vi "uc480_SimpleLive_Memory_Sequence.vi"() -> ()   [LabVIEW 2011]
uses:
  C:/Program Files/Thorlabs/Scientific Imaging/DCx Camera Support/Develop/DotNet/uc480DotNet.dll
  Develop/DotNet/uc480DotNet.dll
panel:
  out "Acquisition":picture
  in  "Active \nAcquisition Buffer":i32 min=0 max=2 step=1
  in  "Active \nOutput Buffer":u32 max=2 step=1
  in  "Num Buffers":i32=2 min=0 max=100 step=1
  out "Output":picture
  in  "Camera ID":i32
  out "Serial Number":string
  out "AOI Height":i32=8
  out "AOI Width":i32=8
  out "Bits/Pixel":i32=8
  out "Error Out":errorcluster caption="error"
  in  "Exit Camera":bool
  in  "Init Camera":bool
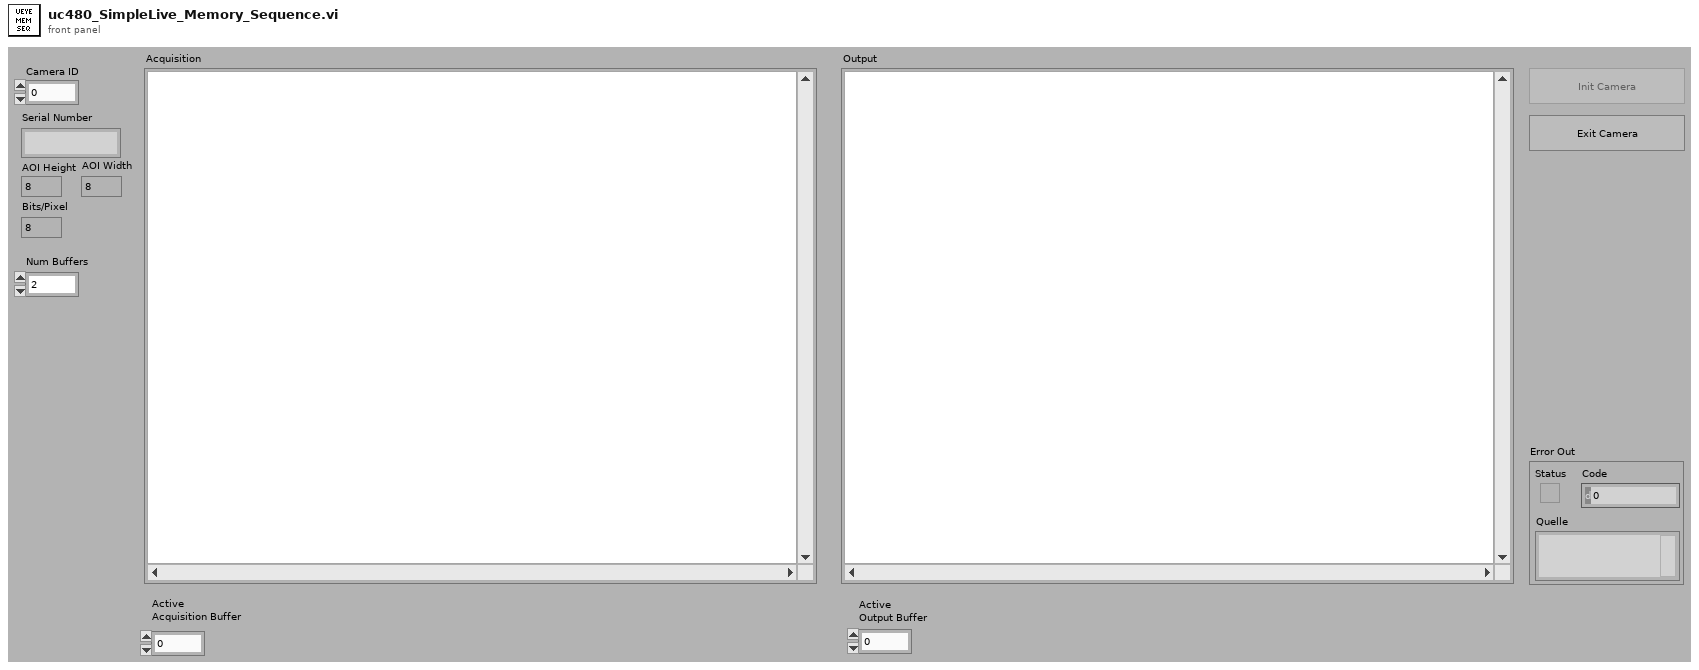
[diagram p1: front panel]
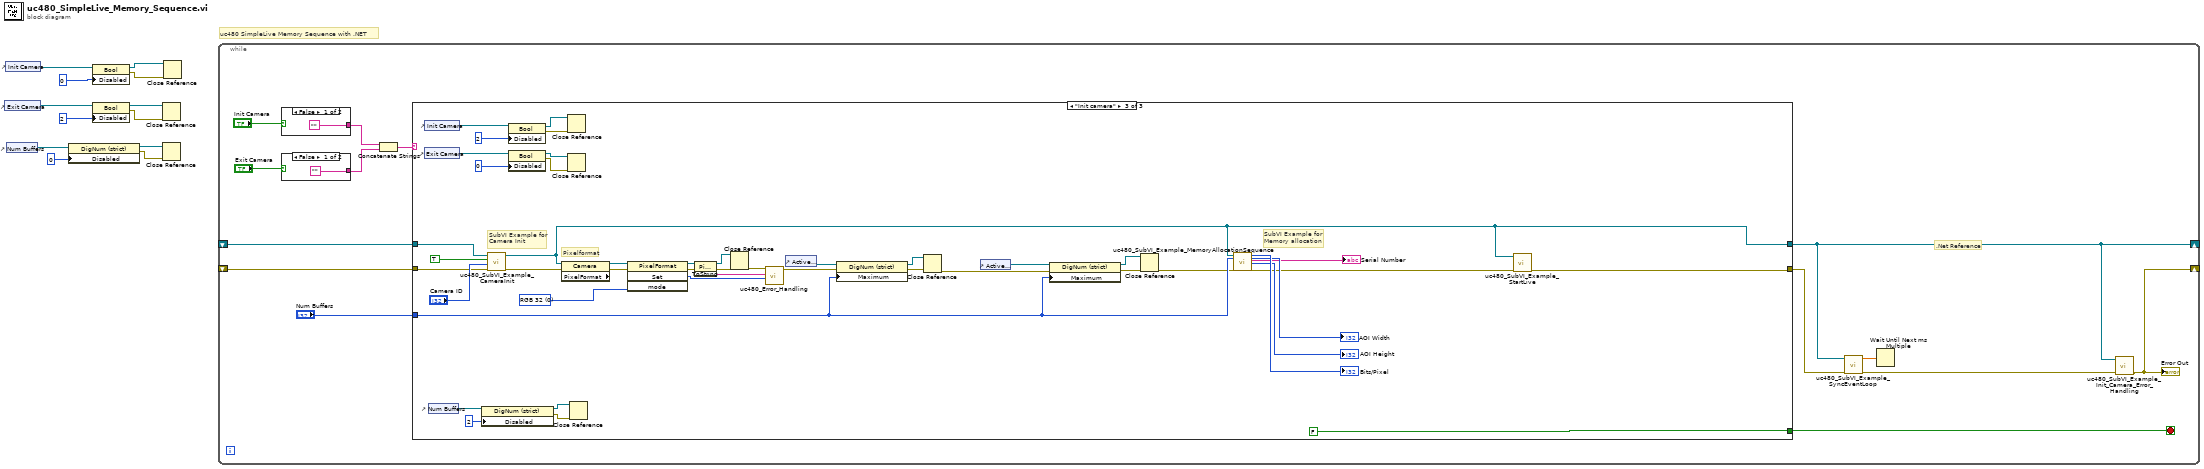
[diagram p0: block diagram]
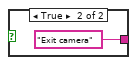
[diagram p2: hidden frame]
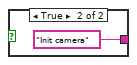
[diagram p3: hidden frame]
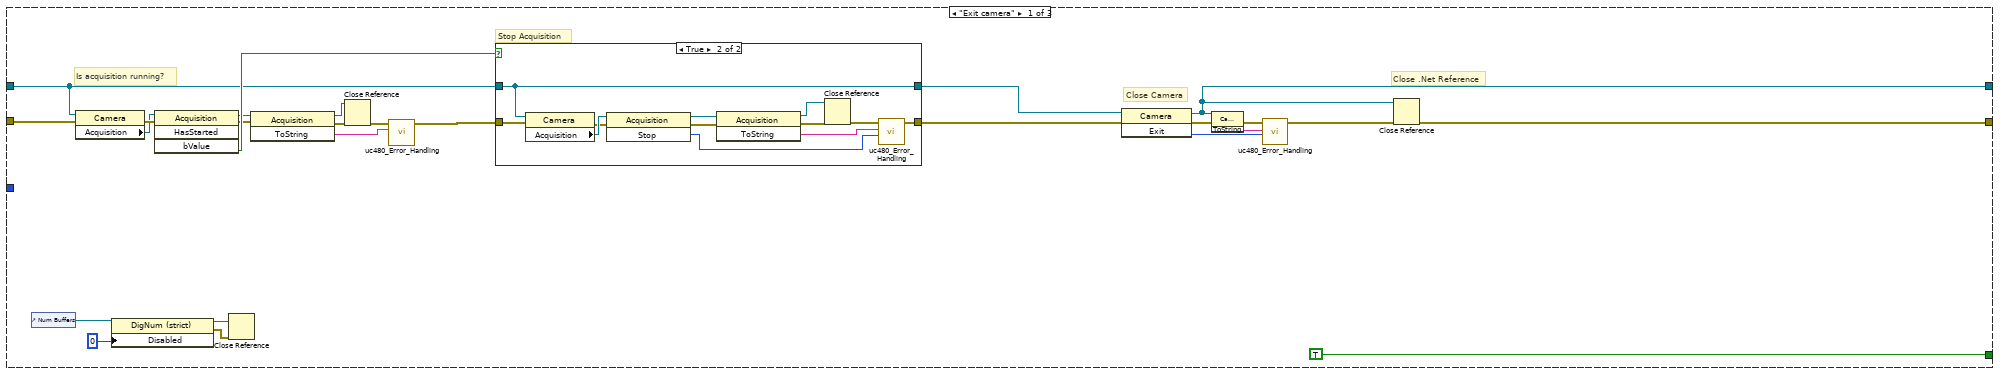
[diagram p4: hidden frame]
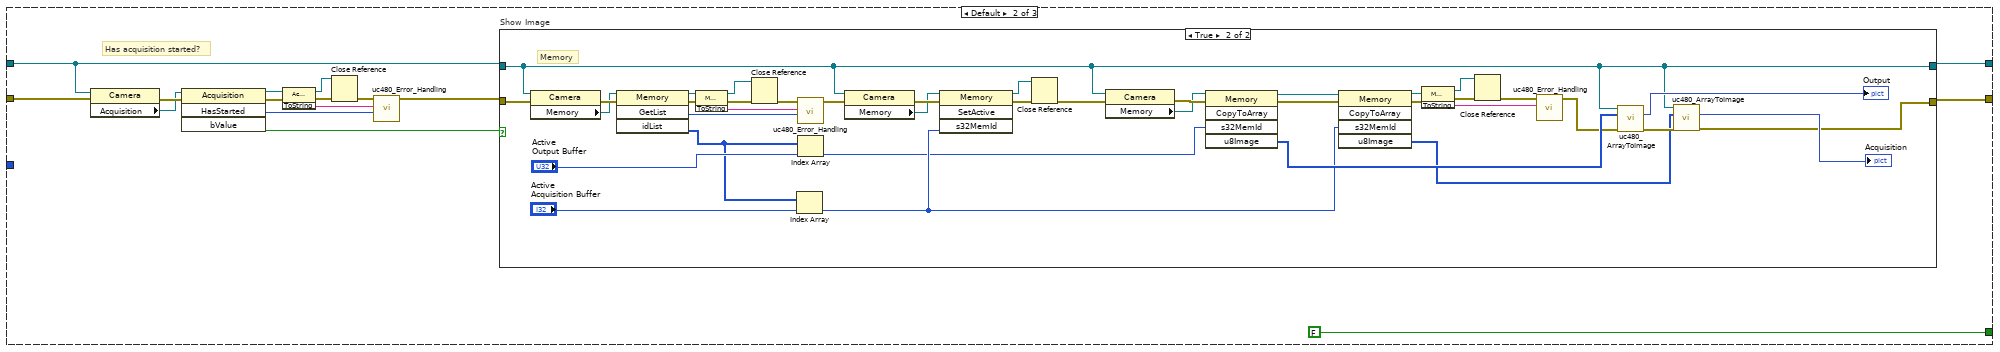
[diagram p6: hidden frame]
diagram:
  # "uc480 SimpleLive Memory Sequence with .NET"
  n1 = control-ref of="Exit Camera"() -> (w9:refnum<vi>)
  n2 = control-ref of="Init Camera"() -> (w11:refnum<vi>)
  n3 = control-ref of="Num Buffers"() -> (w7:refnum<vi>)
  n4 = property class="DigNum (strict)"(reference=w7, "Disabled"=u8 0 ("Deaktiviert")) -> (reference out=w2:refnum<vi>, error out=w1:errorcluster)  [unwired: 1 in]
  n5 = property class="Bool"(reference=w11, "Disabled"=u8 0 ("Deaktiviert")) -> (reference out=w6:refnum<vi>, error out=w5:errorcluster)  [unwired: 1 in]
  n6 = property class="Bool"(reference=w9, "Disabled"=u8 2 ("Deaktiviert")) -> (reference out=w4:refnum<vi>, error out=w3:errorcluster)  [unwired: 1 in]
  n7 = Close Reference ("Close Referenz")(reference=w4, error in (no error)=w3) -> ()  [unwired: 1 out]
  n8 = Close Reference ("Close Referenz")(reference=w2, error in (no error)=w1) -> ()  [unwired: 1 out]
  n9 = Close Reference ("Close Referenz")(reference=w6, error in (no error)=w5) -> ()  [unwired: 1 out]
  n10 = while {
    shift-right: [w19] -> _
    shift-left: _ -> [w21]
    shift-right: [w16] -> _
    shift-left: _ -> [w13]
    stop <- w20 stop-if-true
    # ".Net Reference"
    n11 = case shown="False" "Init Camera" {
      tunnel: ["" "Init camera"] -> w25
      frame False {
      }
      frame True {
      }
    }
    n12 = case shown="False" "Exit Camera" {
      tunnel: ["" "Exit camera"] -> w22
      frame False {
      }
      frame True {
      }
    }
    n13 = Concatenate Strings(w25, w22) -> (w24:string)
    n14 = case shown="\"Init camera\"" w24 {
      tunnel: w13 -> [w40 w75 w164]
      tunnel: w21 -> [w41 w74 w163]
      tunnel: [w49 w77 w143] -> w16
      tunnel: [w50 w76 w144] -> w17
      tunnel: [TRUE FALSE FALSE] -> w20
      tunnel: "Num Buffers" -> [_ _ w153]
      frame "Exit camera" {
        # "Close .Net Reference"
        # "Is acquisition running?"
        # "Stop Acquisition"
        # "Close Camera"
        n15 = control-ref of="Num Buffers"() -> (w36:refnum<vi>)
        n16 = property class="Camera"(reference=w40, error in=w41) -> (error out=w48:errorcluster, "Acquisition"=w47:refnum<k24>)  [unwired: 1 out]
        n17 = property class="DigNum (strict)"(reference=w36, "Disabled"=u8 0 ("Deaktiviert")) -> (reference out=w32:refnum<vi>, error out=w31:errorcluster)  [unwired: 1 in]
        n18 = invoke class="Acquisition" method="HasStarted"(reference=w47, error in=w48) -> (reference out=w42:refnum<k24>, error out=w44:errorcluster, "bValue"=w46:bool)  [unwired: 2 in, 1 out]
        n19 = Close Reference ("Close Referenz")(reference=w32, error in (no error)=w31) -> ()  [unwired: 1 out]
        n20 = invoke class="Acquisition" method="ToString"(reference=w42, error in=w44) -> (reference out=w33:refnum<k24>, error out=w35:errorcluster, "ToString"=w43:string)  [unwired: 1 in]
        n21 = Close Reference(reference=w33, error in (no error)=w35) -> (error out=w34:errorcluster)
        n22 = call "uc480_Error_Handling.vi"("Error String"=w43, "Error In"=w34) -> ("Error Out"=w45:errorcluster)  [unwired: 9 in]
        n23 = case shown="True" w46 {
          tunnel: [w58 w69] -> w38
          tunnel: w45 -> [w58 w70]
          tunnel: w40 -> [w57 w62]
          tunnel: [w57 w62] -> w39
          frame False {
          }
          frame True {
            n24 = property class="Camera"(reference=w62, error in=w70) -> (error out=w66:errorcluster, "Acquisition"=w67:refnum<k24>)  [unwired: 1 out]
            n25 = invoke class="Acquisition" method="Stop"(reference=w67, error in=w66) -> (reference out=w64:refnum<k24>, error out=w65:errorcluster, "Stop"=w63:i32)  [unwired: 1 in]
            n26 = invoke class="Acquisition" method="ToString"(reference=w64, error in=w65) -> (reference out=w59:refnum<k24>, error out=w61:errorcluster, "ToString"=w68:string)  [unwired: 1 in]
            n27 = Close Reference(reference=w59, error in (no error)=w61) -> (error out=w60:errorcluster)
            n28 = call "uc480_Error_Handling.vi"("Error Code"=w63, "Error String"=w68, "Error In"=w60) -> ("Error Out"=w69:errorcluster)  [unwired: 8 in]
          }
        }
        n29 = invoke class="Camera" method="Exit"(reference=w39, error in=w38) -> (reference out=w49:refnum<k24>, error out=w53:errorcluster, "Exit"=w52:i32)  [unwired: 1 in]
        n30 = invoke class="Camera" method="ToString"(reference=w49, error in=w53) -> (error out=w54:errorcluster, "ToString"=w55:string)  [unwired: 1 in, 1 out]
        n31 = call "uc480_Error_Handling.vi"("Error Code"=w52, "Error String"=w55, "Error In"=w54) -> ("Error Out"=w51:errorcluster)  [unwired: 8 in]
        n32 = Close Reference ("Close Referenz")(reference=w49, error in (no error)=w51) -> (error out=w50:errorcluster)
      }
      frame Default {
        # "Has acquisition started?"
        n33 = property class="Camera"(reference=w75, error in=w74) -> (error out=w85:errorcluster, "Acquisition"=w84:refnum<k24>)  [unwired: 1 out]
        n34 = invoke class="Acquisition" method="HasStarted"(reference=w84, error in=w85) -> (reference out=w81:refnum<k24>, error out=w80:errorcluster, "HasStarted"=w79:i32, "bValue"=w83:bool)  [unwired: 2 in]
        n35 = invoke class="Acquisition" method="ToString"(reference=w81, error in=w80) -> (reference out=w71:refnum<k24>, error out=w73:errorcluster, "ToString"=w82:string)  [unwired: 1 in]
        n36 = Close Reference(reference=w71, error in (no error)=w73) -> (error out=w72:errorcluster)
        n37 = call "uc480_Error_Handling.vi"("Error Code"=w79, "Error String"=w82, "Error In"=w72) -> ("Error Out"=w78:errorcluster)  [unwired: 8 in]
        n38 = case "Show Image" shown="True" w83 {
          tunnel: [w88 w99] -> w76
          tunnel: w78 -> [w88 w119]
          tunnel: w75 -> [w87 w101]
          tunnel: [w87 w101] -> w77
          frame False {
          }
          frame True {
            # "Memory"
            n39 = property class="Camera"(reference=w101, error in=w119) -> (error out=w120:errorcluster, "Memory"=w118:refnum<k24>)  [unwired: 1 out]
            n40 = invoke class="Memory" method="GetList"(reference=w118, error in=w120) -> (reference out=w125:refnum<k24>, error out=w124:errorcluster, "GetList"=w126:i32, "idList"=w112:i32[])  [unwired: 2 in]
            n41 = invoke class="Memory" method="ToString"(reference=w125, error in=w124) -> (reference out=w96:refnum<k24>, error out=w98:errorcluster, "ToString"=w123:string)  [unwired: 1 in]
            n42 = Close Reference(reference=w96, error in (no error)=w98) -> (error out=w97:errorcluster)
            n43 = Index Array(array=w112, index="Active \nAcquisition Buffer") -> (element=w108:i32)
            n44 = call "uc480_Error_Handling.vi"("Error Code"=w126, "Error String"=w123, "Error In"=w97) -> ("Error Out"=w115:errorcluster)  [unwired: 8 in]
            n45 = Index Array(array=w112, index="Active \nOutput Buffer") -> (element=w100:i32)
            n46 = property class="Camera"(reference=w101, error in=w115) -> (error out=w114:errorcluster, "Memory"=w113:refnum<k24>)  [unwired: 1 out]
            n47 = invoke class="Memory" method="SetActive"(reference=w113, error in=w114, "s32MemId"=w108) -> (reference out=w93:refnum<k24>, error out=w95:errorcluster)  [unwired: 1 in, 2 out]
            n48 = Close Reference(reference=w93, error in (no error)=w95) -> (error out=w94:errorcluster)
            n49 = property class="Camera"(reference=w101, error in=w94) -> (error out=w122:errorcluster, "Memory"=w110:refnum<k24>)  [unwired: 1 out]
            n50 = invoke class="Memory" method="CopyToArray"(reference=w110, error in=w122, "s32MemId"=w100) -> (reference out=w92:refnum<k24>, error out=w109:errorcluster, "u8Image"=w121:u8[])  [unwired: 2 in, 2 out]
            n51 = invoke class="Memory" method="CopyToArray"(reference=w92, error in=w109, "s32MemId"=w108) -> (reference out=w106:refnum<k24>, error out=w107:errorcluster, "u8Image"=w102:u8[])  [unwired: 2 in, 2 out]
            n52 = invoke class="Memory" method="ToString"(reference=w106, error in=w107) -> (reference out=w89:refnum<k24>, error out=w91:errorcluster, "ToString"=w127:string)  [unwired: 1 in]
            n53 = Close Reference(reference=w89, error in (no error)=w91) -> (error out=w90:errorcluster)
            n54 = call "uc480_Error_Handling.vi"("Error String"=w127, "Error In"=w90) -> ("Error Out"=w117:errorcluster)  [unwired: 9 in]
            n55 = call "uc480_ArrayToImage.vi"("Error In"=w117, "InArray"=w121, ".NET (Reference)"=w101) -> ("Error Out"=w105:errorcluster, "Image"=→"Output":picture)  [unwired: 7 in]
            n56 = call "uc480_ArrayToImage.vi"("Error In"=w105, "InArray"=w102, ".NET (Reference)"=w101) -> ("Error Out"=w99:errorcluster, "Image"=→"Acquisition":picture)  [unwired: 7 in]
          }
        }
      }
      frame "Init camera" {
        w172 = 0 items=["RGB 32"=0, "RGB 24"=1, "Y8 Monochrom"=6] ("Mode")
        # "SubVI Example for \nMemory allocation"
        # "SubVI Example for \nCamera Init"
        # "Pixelformat"
        n57 = control-ref of="Init Camera"() -> (w146:refnum<vi>)
        n58 = control-ref of="Exit Camera"() -> (w148:refnum<vi>)
        n59 = control-ref of="Num Buffers"() -> (w151:refnum<vi>)
        n60 = property class="DigNum (strict)"(reference=w151, "Disabled"=u8 2 ("Deaktiviert")) -> (reference out=w135:refnum<vi>, error out=w134:errorcluster)  [unwired: 1 in]
        n61 = call "uc480_SubVI_Example_CameraInit.vi"("Error In"=w163, "Camera ID"="Camera ID", "Init Camera Flag"=TRUE, ".NET (Reference)"=w164) -> ("Error Out"=w169:errorcluster, ".NET (Reference)"=w143:refnum<k24>)  [unwired: 6 in]
        n62 = property class="Bool"(reference=w146, "Disabled"=u8 2 ("Deaktiviert")) -> (reference out=w139:refnum<vi>, error out=w138:errorcluster)  [unwired: 1 in]
        n63 = property class="Bool"(reference=w148, "Disabled"=u8 0 ("Deaktiviert")) -> (reference out=w137:refnum<vi>, error out=w136:errorcluster)  [unwired: 1 in]
        n64 = property class="Camera"(reference=w143, error in=w169) -> (error out=w170:errorcluster, "PixelFormat"=w171:refnum<k24>)  [unwired: 1 out]
        n65 = Close Reference ("Close Referenz")(reference=w139, error in (no error)=w138) -> ()  [unwired: 1 out]
        n66 = Close Reference ("Close Referenz")(reference=w137, error in (no error)=w136) -> ()  [unwired: 1 out]
        n67 = Close Reference ("Close Referenz")(reference=w135, error in (no error)=w134) -> ()  [unwired: 1 out]
        n68 = invoke class="PixelFormat" method="Set"(reference=w171, error in=w170, "mode"=w172) -> (reference out=w167:refnum<k24>, error out=w160:errorcluster, "Set"=w166:i32)  [unwired: 1 in, 1 out]
        n69 = invoke class="PixelFormat" method="ToString"(reference=w167, error in=w160) -> (reference out=w140:refnum<k24>, error out=w142:errorcluster, "ToString"=w168:string)  [unwired: 1 in]
        n70 = Close Reference(reference=w140, error in (no error)=w142) -> (error out=w141:errorcluster)
        n71 = call "uc480_Error_Handling.vi"("Error Code"=w166, "Error String"=w168, "Error In"=w141) -> ("Error Out"=w152:errorcluster)  [unwired: 8 in]
        n72 = control-ref of="Active \nOutput Buffer"() -> (w154:refnum<vi>)
        n73 = property class="DigNum (strict)"(reference=w154, error in=w152, "Maximum"=w153) -> (reference out=w132:refnum<vi>, error out=w133:errorcluster)
        n74 = Close Reference ("Close Referenz")(reference=w132, error in (no error)=w133) -> (error out=w131:errorcluster)
        n75 = control-ref of="Active \nAcquisition Buffer"() -> (w155:refnum<vi>)
        n76 = property class="DigNum (strict)"(reference=w155, error in=w131, "Maximum"=w153) -> (reference out=w128:refnum<vi>, error out=w130:errorcluster)
        n77 = Close Reference ("Close Referenz")(reference=w128, error in (no error)=w130) -> (error out=w129:errorcluster)
        n78 = call "uc480_SubVI_Example_MemoryAllocationSequence.vi"(".NET (Reference)"=w143, "Num Buffers"=w153, "Fehler (Eingang, kein Fehler)"=w129) -> ("Bits/Pixel 2"=→"Bits/Pixel":i32, "Width"=→"AOI Width":i32, "Serial Number"=→"Serial Number":string, "Height"=→"AOI Height":i32, "Fehler (Ausgang)"=w145:errorcluster)  [unwired: 11 in, 1 out]
        n79 = call "uc480_SubVI_Example_StartLive.vi"("Error"=w145, ".NET (Reference)"=w143) -> ("Error"=w144:errorcluster)  [unwired: 9 in]
      }
    }
    n80 = call "uc480_SubVI_Example_SyncEventLoop.vi"("Error In"=w17, ".NET (Reference)"=w16) -> ("Error Out"=w15:errorcluster, "Synchronize (ms)"=w14:dbl)  [unwired: 8 in]
    n81 = Wait Until Next ms Multiple(millisecond multiple=w14) -> ()  [unwired: 1 out]
    n82 = call "uc480_SubVI_Example_Init_Camera_Error_Handling.vi"("Error In"=w15, ".NET (Reference)"=w16) -> ("Error Out"=w19:errorcluster)  [unwired: 9 in]
    "Error Out" <- w19
  }
